vi "Euler Angles to Rotation Matrix.vi"(1 "euler angles":T2) -> (0 "rotation matrix":T1)   [LabVIEW 2017, in "NI_Kinematics.lvlib"]
doc: "Converts the Z, X, and Z Euler angle values you specify to the corresponding <B>rotation matrix</B>.\n\n<B>.m file:</B> eul2r"
uses:
  <vilib>/robotics/Kinematics/NI_Kinematics.lvlib
  <vilib>/Analysis/Matrix/Datatypes/RealMatrix.ctl
  <vilib>/Analysis/NI_AALPro.lvlib
  <vilib>/Analysis/Matrix/NI_Matrix.lvlib
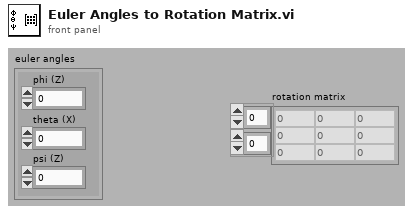
[diagram p1: front panel]
types:
  T1 = typedef "NI_Matrix.lvlib/RealMatrix.ctl" = dbl[][]
  T2 = cluster{"phi (Z)":dbl, "theta (X)":dbl, "psi (Z)":dbl}
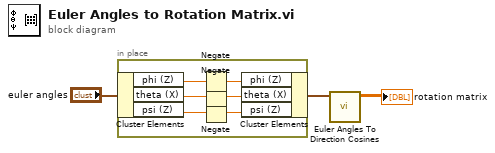
[diagram p0: block diagram]
diagram:
  n1 = in-place {
    n2 = in-place-cluster #1("euler angles") -> ("phi (Z)"=w8:dbl, "theta (X)"=w9:dbl, "psi (Z)"=w7:dbl)
    n3 = Negate(x=w8) -> (-x=w4:dbl)
    n4 = Negate(x=w9) -> (-x=w5:dbl)
    n5 = Negate(x=w7) -> (-x=w6:dbl)
    n6 = in-place-cluster #1("phi (Z)"=w4, "theta (X)"=w5, "psi (Z)"=w6) -> (w3:T2)
  }
  n7 = call <vilib>:"Euler Angles To Direction Cosines.vi"("Euler Angles"=w3) -> ("Direction Cosines"=→"rotation matrix":dbl[][])  [unwired: 9 in, 1 out]
